vi "Add Channel right-click menu.vi"(8 "error in (no error)":errorcluster, 11 "Node Ptr":u64 format="%.0x") -> (0 "error out":errorcluster)   [LabVIEW 2016, in "UDP Sender System Explorer.lvlib"]
uses:
  System Explorer/UDP Sender System Explorer.lvlib
  <vilib>/NI Veristand/Custom Device API/Custom Device Channel.ctl
  <vilib>/NI Veristand/Custom Device API/Custom Device Channel Type.ctl
  <vilib>/NI Veristand/Custom Device API/Custom Device API.lvlib
panel:
  in  "OK":bool
  in  "Channel":T1
  in  "Channel Name":string
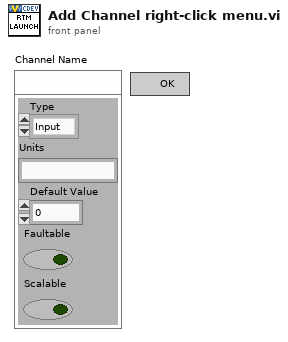
[diagram p1: front panel]
types:
  T1 = typedef "Custom Device API.lvlib/Custom Device Channel.ctl" = cluster{"Type":T2, "Units":string, "Default Value":dbl, "Faultable":bool, "Scalable":bool}
  T2 = typedef "Custom Device API.lvlib/Custom Device Channel Type.ctl" = enum16{"Input", "Output"}
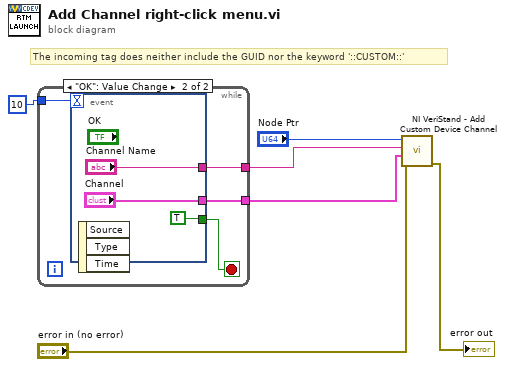
[diagram p0: block diagram]
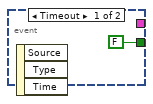
[diagram p2: hidden frame]
diagram:
  # "The incoming tag does neither include the GUID nor the keyword '::CUSTOM::'"
  n1 = while {
    tunnel: [w9] -> w5
    tunnel: [w8] -> w4
    tunnel: 10 -> [w7]
    stop <- w10 stop-if-true
    n2 = event shown="[1] \"OK\": Value Change" {
      selector: _ -> [_ _]
      dyn-events: _ -> [_ _]
      timeout: w7 -> [_ _]
      tunnel: [FALSE TRUE] -> w10
      tunnel: [_ "Channel Name"] -> w9
      tunnel: [_ "Channel"] -> w8
      event Timeout {
        n3 = event-data() -> ()  [unwired: 1 in, 3 out]
      }
      event "OK": Value Change {
        n4 = event-data() -> ()  [unwired: 1 in, 3 out]
      }
    }
  }
  n5 = call <vilib>:"NI VeriStand - Add Custom Device Channel.vi"("error in (no error)"="error in (no error)", "Channel"=w4, "Channel Name"=w5, "Parent Ref in"="Node Ptr") -> ("error out"=→"error out":errorcluster)  [unwired: 4 in, 3 out]
